vi "03_inputPacketParsing.vi"(11 "string":string) -> (0 "TrigTimer, s":dbl, 1 "Service state":cluster{u8, u8}, 2 "DAC state":cluster{dbl, dbl, dbl, dbl}, 3 "Voltage":cluster{dbl, dbl, dbl, dbl}, 5 "CurrentError":bool)   [LabVIEW 2017]
panel:
  out "FirstByte":bool
  out "Service Byte":u8
  out "Knob Byte":u8
  out "DAC2volt, V":dbl format="%.3f"
  out "DAC1volt, V":dbl format="%.3f"
  out "DAC2cur, mA":dbl format="%.5f"
  out "DAC1cur, mA":dbl format="%.5f"
  out "Ch4, V":dbl format="%.3f"
  out "Ch3, V":dbl format="%.3f"
  out "Ch2, V":dbl format="%.3f"
  out "Ch1, V":dbl format="%.3f"
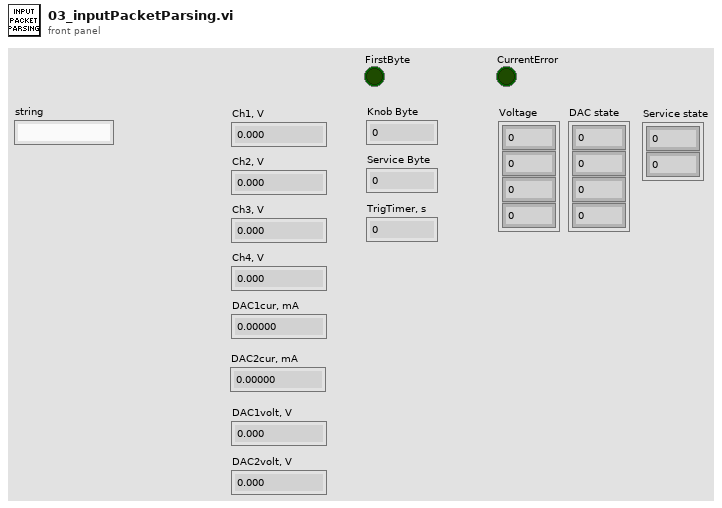
[diagram p1: front panel]
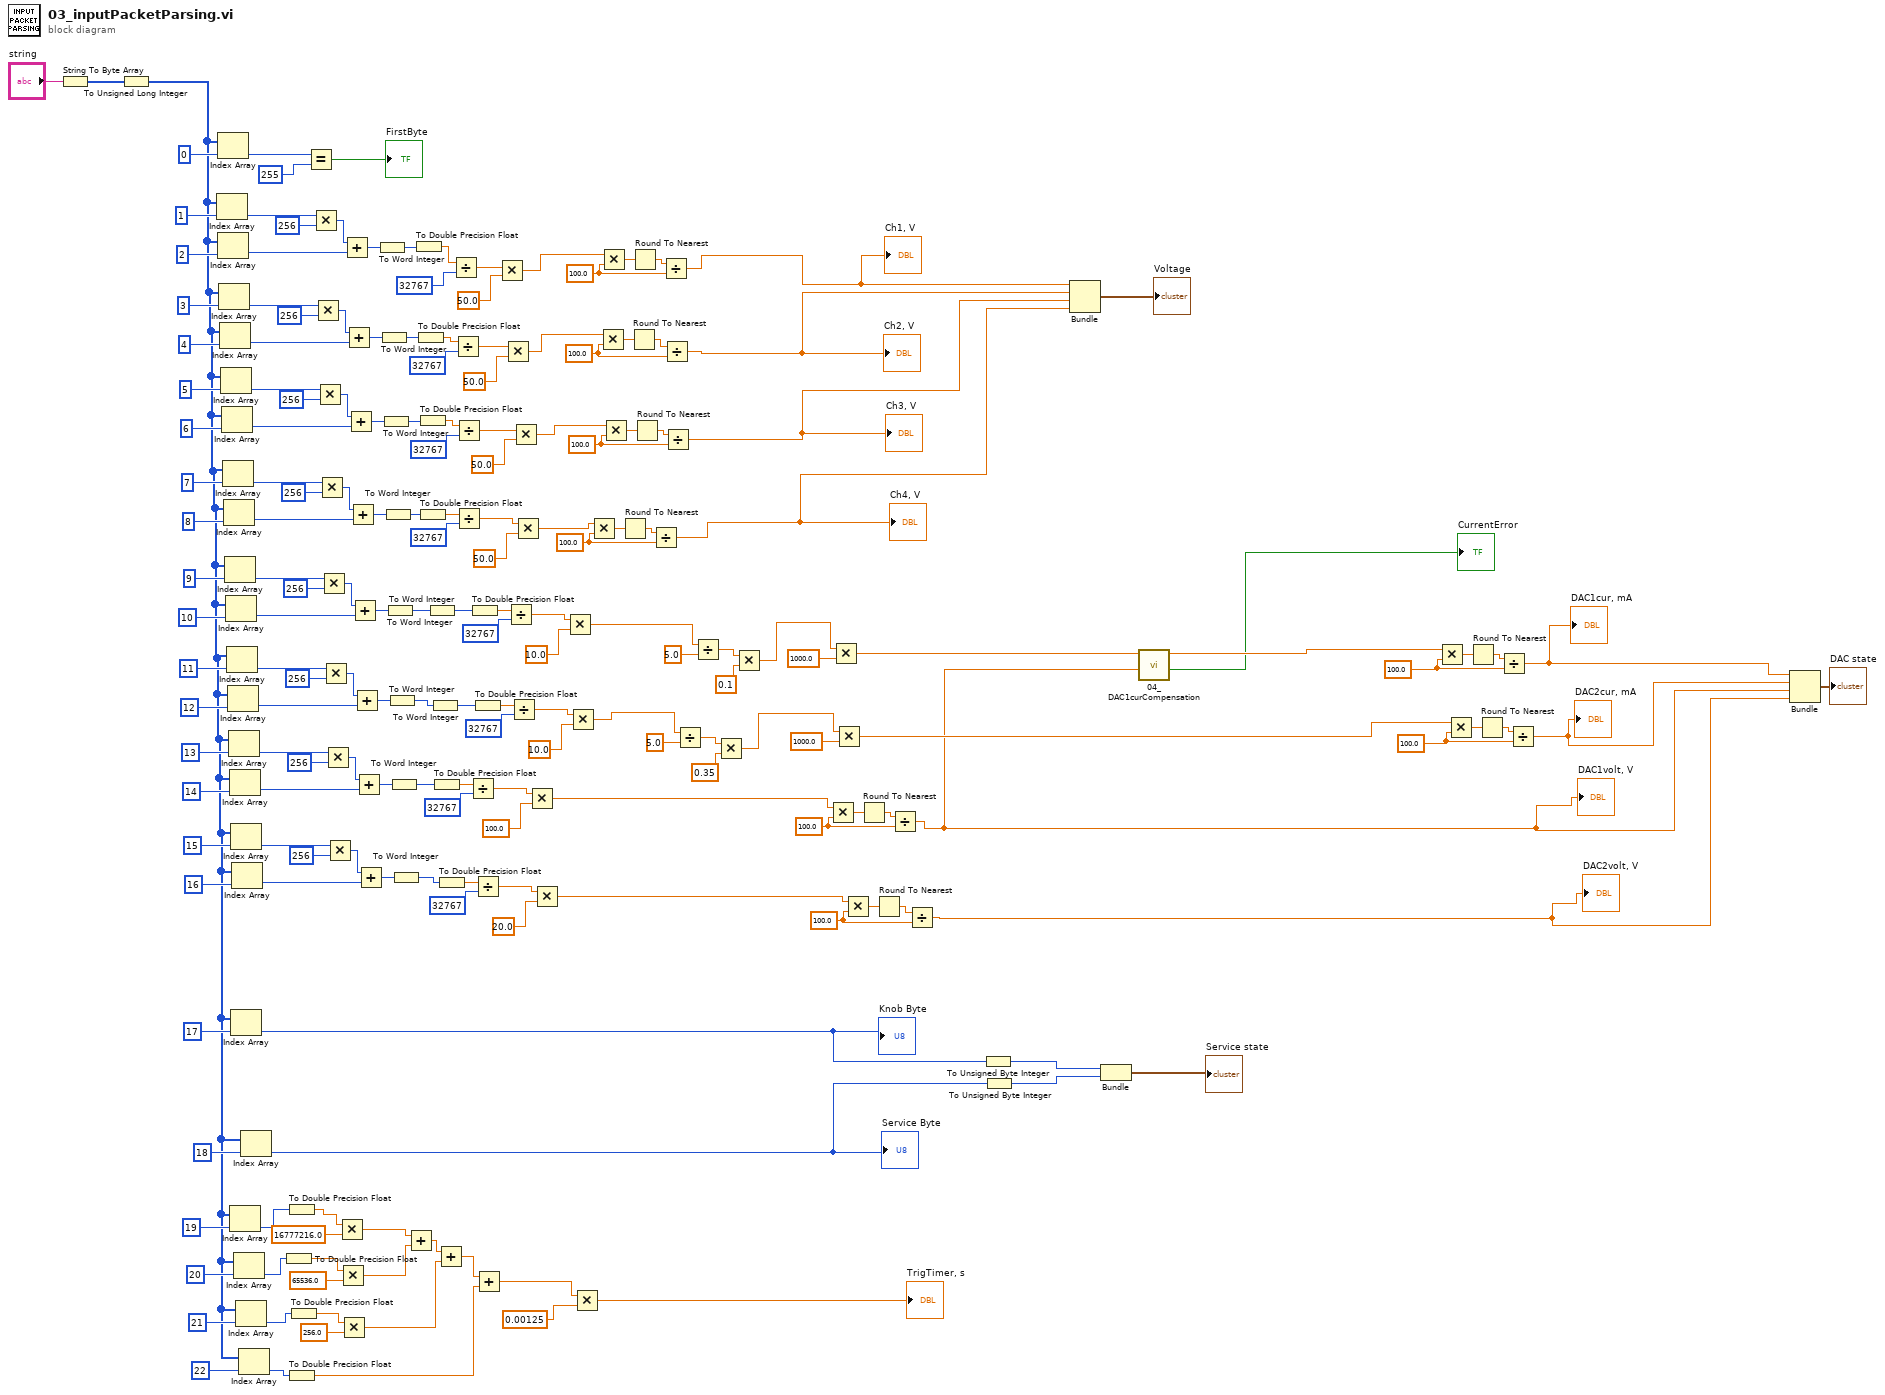
[diagram p0: block diagram]
diagram:
  w15 = 100.0
  w18 = 100.0
  w23 = 100.0
  w27 = 100.0
  w32 = 100.0
  w37 = 100.0
  w42 = 100.0
  w47 = 100.0
  n1 = String To Byte Array(string="string") -> (unsigned byte array=w50:u8[])
  n2 = To Unsigned Long Integer(number=w50) -> (unsigned 32bit integer=w49:u32[])
  n3 = Index Array(array=w49, index=1) -> (element=w189:u32)
  n4 = Index Array(array=w49, index=0) -> (element=w55:u32)
  n5 = Index Array(array=w49, index=2) -> (element=w186:u32)
  n6 = Index Array(array=w49, index=3) -> (element=w182:u32)
  n7 = Index Array(array=w49, index=4) -> (element=w179:u32)
  n8 = Index Array(array=w49, index=5) -> (element=w175:u32)
  n9 = Index Array(array=w49, index=6) -> (element=w172:u32)
  n10 = Index Array(array=w49, index=7) -> (element=w168:u32)
  n11 = Index Array(array=w49, index=8) -> (element=w165:u32)
  n12 = Index Array(array=w49, index=9) -> (element=w161:u32)
  n13 = Index Array(array=w49, index=10) -> (element=w158:u32)
  n14 = Index Array(array=w49, index=11) -> (element=w154:u32)
  n15 = Index Array(array=w49, index=12) -> (element=w151:u32)
  n16 = Index Array(array=w49, index=13) -> (element=w147:u32)
  n17 = Index Array(array=w49, index=14) -> (element=w144:u32)
  n18 = Index Array(array=w49, index=19) -> (element=w66:u32)
  n19 = Index Array(array=w49, index=15) -> (element=w140:u32)
  n20 = Index Array(array=w49, index=17) -> (element=w3:u32)
  "Knob Byte" <- w3
  n21 = Index Array(array=w49, index=16) -> (element=w137:u32)
  n22 = Index Array(array=w49, index=20) -> (element=w67:u32)
  n23 = Index Array(array=w49, index=21) -> (element=w70:u32)
  n24 = Index Array(array=w49, index=22) -> (element=w72:u32)
  n25 = Index Array(array=w49, index=18) -> (element=w4:u32)
  "Service Byte" <- w4
  n26 = To Double Precision Float(number=w67) -> (double precision float=w68:dbl)
  n27 = To Double Precision Float(number=w66) -> (double precision float=w65:dbl)
  n28 = To Double Precision Float(number=w72) -> (double precision float=w71:dbl)
  n29 = To Double Precision Float(number=w70) -> (double precision float=w69:dbl)
  n30 = Equal?(x=w55, y=u32 255) -> (x = y?=→"FirstByte":bool)
  n31 = Multiply(x=w189, y=u32 256) -> (x*y=w187:u32)
  n32 = Multiply(x=w182, y=u32 256) -> (x*y=w180:u32)
  n33 = Multiply(x=w175, y=u32 256) -> (x*y=w173:u32)
  n34 = Multiply(x=w168, y=u32 256) -> (x*y=w166:u32)
  n35 = Multiply(x=w161, y=u32 256) -> (x*y=w159:u32)
  n36 = Multiply(x=w154, y=u32 256) -> (x*y=w152:u32)
  n37 = Multiply(x=w147, y=u32 256) -> (x*y=w145:u32)
  n38 = Multiply(x=w140, y=u32 256) -> (x*y=w138:u32)
  n39 = Multiply(x=w65, y=16777216.0) -> (x*y=w80:dbl)
  n40 = Multiply(x=w68, y=65536.0) -> (x*y=w79:dbl)
  n41 = Multiply(x=w69, y=256.0) -> (x*y=w77:dbl)
  n42 = Add(x=w187, y=w186) -> (x+y=w185:u32)
  n43 = Add(x=w180, y=w179) -> (x+y=w178:u32)
  n44 = Add(x=w173, y=w172) -> (x+y=w171:u32)
  n45 = Add(x=w166, y=w165) -> (x+y=w164:u32)
  n46 = Add(x=w159, y=w158) -> (x+y=w157:u32)
  n47 = Add(x=w152, y=w151) -> (x+y=w150:u32)
  n48 = Add(x=w145, y=w144) -> (x+y=w143:u32)
  n49 = Add(x=w138, y=w137) -> (x+y=w136:u32)
  n50 = To Word Integer(number=w185) -> (16bit integer=w116:i16)
  n51 = To Word Integer(number=w178) -> (16bit integer=w126:i16)
  n52 = To Word Integer(number=w171) -> (16bit integer=w129:i16)
  n53 = To Word Integer(number=w164) -> (16bit integer=w130:i16)
  n54 = To Word Integer(number=w157) -> (16bit integer=w93:i16)
  n55 = To Word Integer(number=w150) -> (16bit integer=w94:i16)
  n56 = To Word Integer(number=w143) -> (16bit integer=w106:i16)
  n57 = To Word Integer(number=w136) -> (16bit integer=w105:i16)
  n58 = Add(x=w80, y=w79) -> (x+y=w78:dbl)
  n59 = To Double Precision Float(number=w116) -> (double precision float=w125:dbl)
  n60 = To Double Precision Float(number=w126) -> (double precision float=w127:dbl)
  n61 = To Double Precision Float(number=w129) -> (double precision float=w128:dbl)
  n62 = To Double Precision Float(number=w130) -> (double precision float=w131:dbl)
  n63 = To Word Integer(number=w93) -> (16bit integer=w100:i16)
  n64 = To Word Integer(number=w94) -> (16bit integer=w95:i16)
  n65 = To Double Precision Float(number=w106) -> (double precision float=w109:dbl)
  n66 = Add(x=w78, y=w77) -> (x+y=w76:dbl)
  n67 = To Double Precision Float(number=w105) -> (double precision float=w113:dbl)
  n68 = Divide(x=w125, y=i16 32767) -> (x/y=w124:dbl)
  n69 = Divide(x=w127, y=i16 32767) -> (x/y=w117:dbl)
  n70 = Divide(x=w128, y=i16 32767) -> (x/y=w118:dbl)
  n71 = Divide(x=w131, y=i16 32767) -> (x/y=w119:dbl)
  n72 = Divide(x=w109, y=i16 32767) -> (x/y=w107:dbl)
  n73 = To Double Precision Float(number=w100) -> (double precision float=w103:dbl)
  n74 = To Double Precision Float(number=w95) -> (double precision float=w98:dbl)
  n75 = Divide(x=w113, y=i16 32767) -> (x/y=w111:dbl)
  n76 = Add(x=w76, y=w71) -> (x+y=w58:dbl)
  n77 = Multiply(x=w124, y=50.0) -> (x*y=w43:dbl)
  n78 = Multiply(x=w117, y=50.0) -> (x*y=w38:dbl)
  n79 = Divide(x=w103, y=i16 32767) -> (x/y=w101:dbl)
  n80 = Divide(x=w98, y=i16 32767) -> (x/y=w96:dbl)
  n81 = Multiply(x=w118, y=50.0) -> (x*y=w33:dbl)
  n82 = Multiply(x=w119, y=50.0) -> (x*y=w28:dbl)
  n83 = Multiply(x=w107, y=100.0) -> (x*y=w10:dbl)
  n84 = Multiply(x=w111, y=20.0) -> (x*y=w11:dbl)
  n85 = Multiply(x=w101, y=10.0) -> (x*y=w85:dbl)
  n86 = Multiply(x=w96, y=10.0) -> (x*y=w89:dbl)
  n87 = Multiply(x=w58, y=0.00125) -> (x*y=→"TrigTimer, s":dbl)
  n88 = Multiply(x=w28, y=w32) -> (x*y=w31:dbl)
  n89 = Multiply(x=w38, y=w42) -> (x*y=w41:dbl)
  n90 = Multiply(x=w43, y=w47) -> (x*y=w46:dbl)
  n91 = Multiply(x=w33, y=w37) -> (x*y=w36:dbl)
  n92 = Round To Nearest(number=w31) -> (nearest integer value=w30:dbl)
  n93 = Round To Nearest(number=w41) -> (nearest integer value=w40:dbl)
  n94 = Round To Nearest(number=w46) -> (nearest integer value=w45:dbl)
  n95 = Round To Nearest(number=w36) -> (nearest integer value=w35:dbl)
  n96 = Divide(x=w30, y=w32) -> (x/y=w29:dbl)
  "Ch4, V" <- w29
  n97 = Divide(x=w45, y=w47) -> (x/y=w44:dbl)
  "Ch1, V" <- w44
  n98 = Divide(x=w40, y=w42) -> (x/y=w39:dbl)
  "Ch2, V" <- w39
  n99 = Divide(x=w35, y=w37) -> (x/y=w34:dbl)
  "Ch3, V" <- w34
  n100 = Divide(x=w89, y=5.0) -> (x/y=w90:dbl)
  n101 = Divide(x=w85, y=5.0) -> (x/y=w86:dbl)
  n102 = Multiply(x=w90, y=0.35) -> (x*y=w60:dbl)
  n103 = Multiply(x=w86, y=0.1) -> (x*y=w61:dbl)
  n104 = Multiply(x=w10, y=w18) -> (x*y=w17:dbl)
  n105 = Multiply(x=w61, y=1000.0) -> (x*y=w8:dbl)
  n106 = Multiply(x=w60, y=1000.0) -> (x*y=w19:dbl)
  n107 = Multiply(x=w11, y=w15) -> (x*y=w14:dbl)
  n108 = Round To Nearest(number=w17) -> (nearest integer value=w16:dbl)
  n109 = Round To Nearest(number=w14) -> (nearest integer value=w13:dbl)
  n110 = Divide(x=w16, y=w18) -> (x/y=w9:dbl)
  "DAC1volt, V" <- w9
  n111 = Divide(x=w13, y=w15) -> (x/y=w12:dbl)
  "DAC2volt, V" <- w12
  n112 = To Unsigned Byte Integer(number=w3) -> (unsigned 8bit integer=w6:u8)
  n113 = To Unsigned Byte Integer(number=w4) -> (unsigned 8bit integer=w5:u8)
  n114 = Bundle(w44, w39, w34, w29) -> (→"Voltage":cluster{dbl, dbl, dbl, dbl})  [unwired: 1 in]
  n115 = Bundle(w6, w5) -> (→"Service state":cluster{u8, u8})  [unwired: 1 in]
  n116 = call "04_DAC1curCompensation.vi"("DAC1volt, V"=w9, "DAC1curIN, mA"=w8) -> ("CurrentError"=→"CurrentError":bool, "DAC1curOUT, mA"=w7:dbl)  [unwired: 8 in]
  n117 = Multiply(x=w7, y=w27) -> (x*y=w26:dbl)
  n118 = Multiply(x=w19, y=w23) -> (x*y=w22:dbl)
  n119 = Round To Nearest(number=w26) -> (nearest integer value=w25:dbl)
  n120 = Round To Nearest(number=w22) -> (nearest integer value=w21:dbl)
  n121 = Divide(x=w25, y=w27) -> (x/y=w24:dbl)
  "DAC1cur, mA" <- w24
  n122 = Divide(x=w21, y=w23) -> (x/y=w20:dbl)
  "DAC2cur, mA" <- w20
  n123 = Bundle(w24, w20, w9, w12) -> (→"DAC state":cluster{dbl, dbl, dbl, dbl})  [unwired: 1 in]
